vi "2_6.vi"() -> ()   [LabVIEW 2015]
panel:
  out "Replace String":string
  out "String Subset":string
  out "Lower String":string
  out "Trimmed String":string
  out "Upper string":string
  out "Result String":string
  out "After String":string
  out "Match String":string
  in  "A":string
  out "Before string":string
  in  "B":string
  in  "Unit":string
  in  "C":string
  in  "Volatge meter":dbl(knob) scale=0.0..10.0
  in  "Current meter":dbl(knob) scale=0.0..10.0
  out "String out":string
  out "Date/Time":string
  out "Length":i32
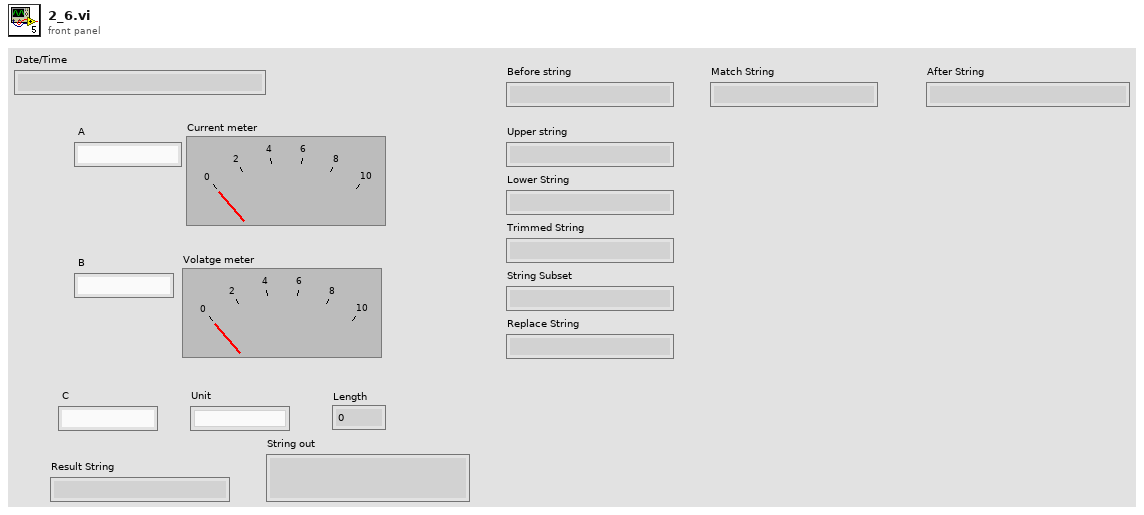
[diagram p1: front panel]
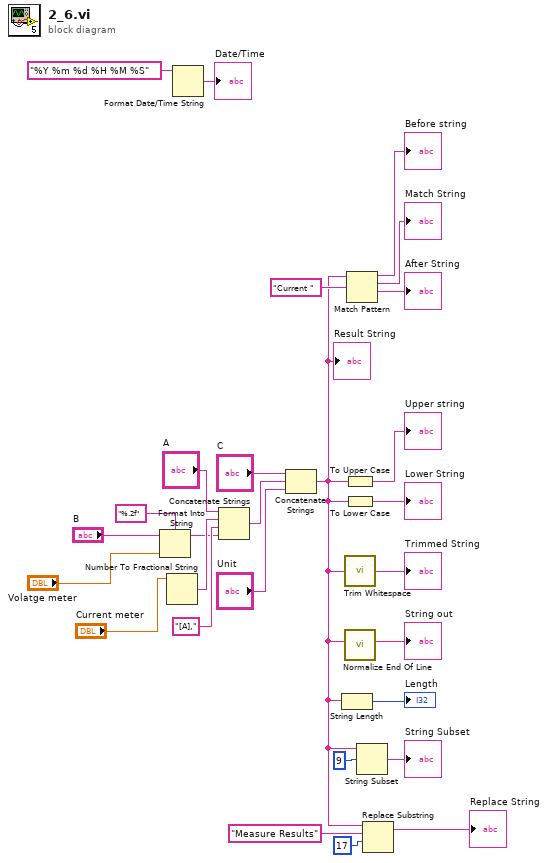
[diagram p0: block diagram]
diagram:
  n1 = Format Into String(format string="%.2f", initial string="B", "Volatge meter") -> (resulting string=w19:string)  [unwired: 1 in, 1 out]
  n2 = Number To Fractional String(number="Current meter") -> (F-format string=w22:string)  [unwired: 3 in]
  n3 = Format Date/Time String(time format string (%c)="%Y %m %d %H %M %S") -> (date/time string=→"Date/Time":string)  [unwired: 2 in]
  n4 = Concatenate Strings("A", w22, "[A]," ("string"), w19) -> (w25:string)
  n5 = Concatenate Strings("C", w25, "Unit") -> (w1:string)
  "Result String" <- w1
  n6 = String Length(string=w1) -> (length=→"Length":i32)
  n7 = To Upper Case(1:w1) -> (0:→"Upper string":string)
  n8 = To Lower Case(string=w1) -> (all lower case string=→"Lower String":string)
  n9 = call <vilib>:"Trim Whitespace.vi"("string"=w1) -> ("trimmed string"=→"Trimmed String":string)  [unwired: 1 in]
  n10 = call <vilib>:"Normalize End Of Line.vi"("string in"=w1) -> ("string out"=→"String out":string)  [unwired: 7 in]
  n11 = Match Pattern(string=w1, regular expression="Current ") -> (before substring=→"Before string":string, match substring=→"Match String":string, after substring=→"After String":string)  [unwired: 1 in, 1 out]
  n12 = String Subset(string=w1, offset (0)=9) -> (substring=→"String Subset":string)  [unwired: 1 in]
  n13 = Replace Substring(3:17 ("offset (0)"), 4:"Measure Results" ("substring (\"\")"), 5:w1) -> (1:→"Replace String":string)  [unwired: 1 in, 1 out]
